vi "ELVIS III v1.0 Close DIO.vi"(8 "error in (no error)":errorcluster, 10 "DIO Channel List":T3, 11 "myRIO Ref In":T1) -> (0 "error out":errorcluster)   [LabVIEW 2021]
uses:
  <vilib>/myRIO/Common/Instrument Driver Framework/myRIO v1.0/DIO/typedefs/DIO Channels List.ctl
  <vilib>/myRIO/Common/Instrument Driver Framework/myRIO v1.0/DIO/typedefs/DIO Channels Enum.ctl
  <vilib>/myRIO/Common/Instrument Driver Framework/Utilities/typedefs/myRIO v1.0 Reference.ctl
  <vilib>/myRIO/Common/Instrument Driver Framework/Utilities/typedefs/Generic FPGA Reference.ctl
  <vilib>/myRIO/Common/Instrument Driver Framework/ELVIS III v1.0/DIO/vis/ELVIS III v1.0 Build MUX Configuration DIO.vi
  <vilib>/myRIO/Common/Instrument Driver Framework/ELVIS III v1.0/Resource Manager/vis/ELVIS III v1.0 Create Configuration List.vi
  <vilib>/myRIO/Common/Instrument Driver Framework/ELVIS III v1.0/Resource Manager/vis/ELVIS III v1.0 Configure IO.vi
  <vilib>/myRIO/Common/Instrument Driver Framework/ELVIS III v1.0/Resource Manager/vis/ELVIS III v1.0 Unreserve Channel List.vi
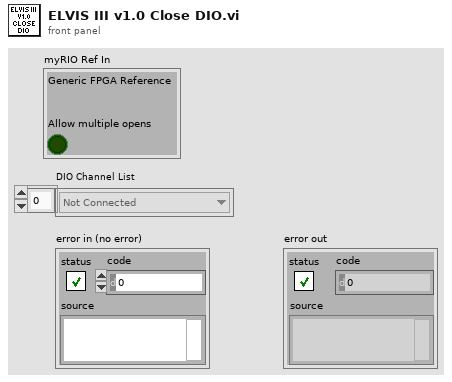
[diagram p1: front panel]
types:
  T1 = typedef "myRIO v1.0 Reference.ctl" = cluster{"Generic FPGA Reference":T2, "Allow multiple opens":bool}
  T2 = typedef "Generic FPGA Reference.ctl" = refnum<k20>
  T3 = typedef "DIO Channels List.ctl" = T4[]
  T4 = typedef "DIO Channels Enum.ctl" = enum16{"Not Connected", "C/DIO0", "C/DIO1", "C/DIO2", "C/DIO3", "C/DIO4", "C/DIO5", "C/DIO6", "C/DIO7", "A/DIO0", "A/DIO1", "A/DIO2", "A/DIO3", "A/DIO4", "A/DIO5", "A/DIO6", "A/DIO7", "A/DIO8", "A/DIO9", "A/DIO10", "A/DIO11", "A/DIO12", "A/DIO13", "A/DIO14", "A/DIO15", "A/DIO16", "A/DIO17", "A/DIO18", "A/DIO19", "B/DIO0", "B/DIO1", "B/DIO2", "B/DIO3", "B/DIO4", "B/DIO5", "B/DIO6", "B/DIO7", "B/DIO8", "B/DIO9", "B/DIO10", "B/DIO11", "B/DIO12", "B/DIO13", "B/DIO14", "B/DIO15", "B/DIO16", "B/DIO17", "B/DIO18", "B/DIO19", "LED0", "LED1", "LED2", "LED3", "Button0", "DIO/DIO0", "DIO/DIO1", "DIO/DIO2", "DIO/DIO3", "DIO/DIO4", "DIO/DIO5", "DIO/DIO6", "DIO/DIO7", "DIO/DIO8", "DIO/DIO9", "SPI/CS0", "SPI/CS1", "SPI/CS2", "SPI/CS3", "LED RADIO (Green)", "LED RADIO (Red)", "LED COMM (Green)", "LED COMM (Red)", "LED MODE (Green)", "LED MODE (Red)"}
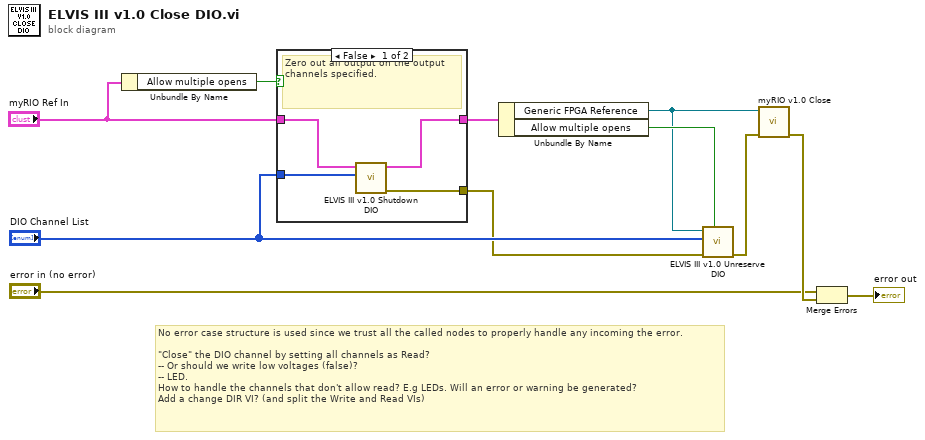
[diagram p0: block diagram]
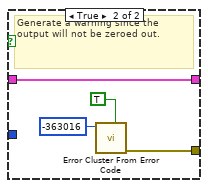
[diagram p2: hidden frame]
diagram:
  # "No error case structure is used since we trust all the called nodes to properly handle any incoming the error.\n\n\"Close\" the DIO channel by setting all channels as Read?\n-- Or should we write low voltages (false)?\n-- LED.\nHow to handle the channels that don't allow read? E.g LEDs. Will an error or warning be generated?\nAdd a change DIR VI? (and split the Write and Read VIs)"
  n1 = Unbundle By Name("myRIO Ref In") -> ("Allow multiple opens"=w5:bool)
  n2 = case shown="False" w5 {
    tunnel: "myRIO Ref In" -> [w15 w19]
    tunnel: [w14 w19] -> w7
    tunnel: "DIO Channel List" -> [w13 _]
    tunnel: [w12 w16] -> w1
    frame False {
      # "Zero out all output on the output channels specified."
      n3 = call <vilib>:"ELVIS III v1.0 Shutdown DIO.vi"("Channel List"=w13, "myRIO Ref In"=w15) -> ("error out"=w12:errorcluster, "myRIO Ref Out"=w14:T1)  [unwired: 8 in]
    }
    frame True {
      # "Generate a warning since the output will not be zeroed out."
      n4 = call <vilib>:"Error Cluster From Error Code.vi"("is warning? (False)"=TRUE, "error code (0)"=-363016) -> ("error out"=w16:errorcluster)  [unwired: 7 in]
    }
  }
  n5 = Unbundle By Name(w7) -> ("Generic FPGA Reference"=w8:T2, "Allow multiple opens"=w9:bool)
  n6 = call <vilib>:"ELVIS III v1.0 Unreserve DIO.vi"("Allow multiple opens?"=w9, "error in (no error)"=w1, "DIO Channel List"="DIO Channel List", "myRIO FPGA Ref In"=w8) -> ("error out"=w11:errorcluster)  [unwired: 7 in]
  n7 = call <vilib>:"myRIO v1.0 Close.vi"("error in (no error)"=w11, "myRIO FPGA Ref In"=w8) -> ("error out"=w10:errorcluster)  [unwired: 9 in]
  n8 = Merge Errors("error in (no error)", w10) -> (→"error out":errorcluster)
